vi "Global.vi"() -> ()   [LabVIEW 2015]
panel:
  in  "停止":bool=TRUE
  in  "被测通道数":i32
  in  "原始记录保存路径":path
  in  "原始记录模板路径":path
  in  "方向选择":string(combo)="Z向"
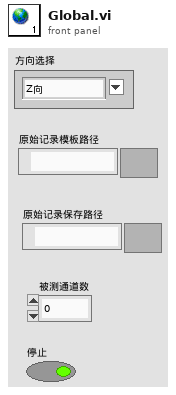
[diagram p1: front panel]
diagram:
